vi "send_manipulatorMultiJump-v02.vi"(0 "daq_ao 2":tag="Dev1/ao1", 1 "Duration (s)":dbl, 2 "controls array in":refnum<vi>[](array[refnum]), 3 "Sample Freq (Hz)":dbl min=0.0 max=40000.0, 4 "Delay":dbl, 5 "Position Dwell Time (s)":dbl[](array[numeric]), 6 "daq_ai":tag="Dev1/ai0:1", 8 "Use Current Position for Start Pos?":bool, 9 "Number of Replicates":i16=1 min=1 max=10, 10 "Start Position":T4(ring)=enum."Jumper Position C", 11 "common cluster":T5, 12 "Jump Position Array":T3(array[ring]), 13 "error in":errorcluster) -> (14 "output cluster":T1, 16 "control array out":refnum<vi>[](array[refnum]), 17 "protcol waveform":waveform(dbl)(graph), 18 "error out":errorcluster, 19 "protcol response":waveform(dbl)[](graph) caption="jumptestMonitor")   [LabVIEW 2019]
uses:
  multipatch/controls/multipatch_common_controls_v4.ctl
  machine_vision/controls/transform_cluster_actuator.ctl
  machine_vision/coordinate model vis/transform_properties_actuators.ctl
  pipette cleaning/pressure box/cleaning_soft/controls/actuator_cluster.ctl
  pipette cleaning/pressure box/cleaning_soft/controls/actuator_type.ctl
  pipette cleaning/pressure box/cleaning_soft/controls/pressure_box_control.ctl
  pipette cleaning/pressure box/cleaning_soft/controls/pressure_box_type.ctl
  controls/NH_method.ctl
  <vilib>/measure/NI_MABase.lvlib
panel:
  out "PositionClusterArray":T2(array[cluster])
  in  "Jump Filter Freq (Hz)":dbl=20.0 min=0.0 max=40000.0
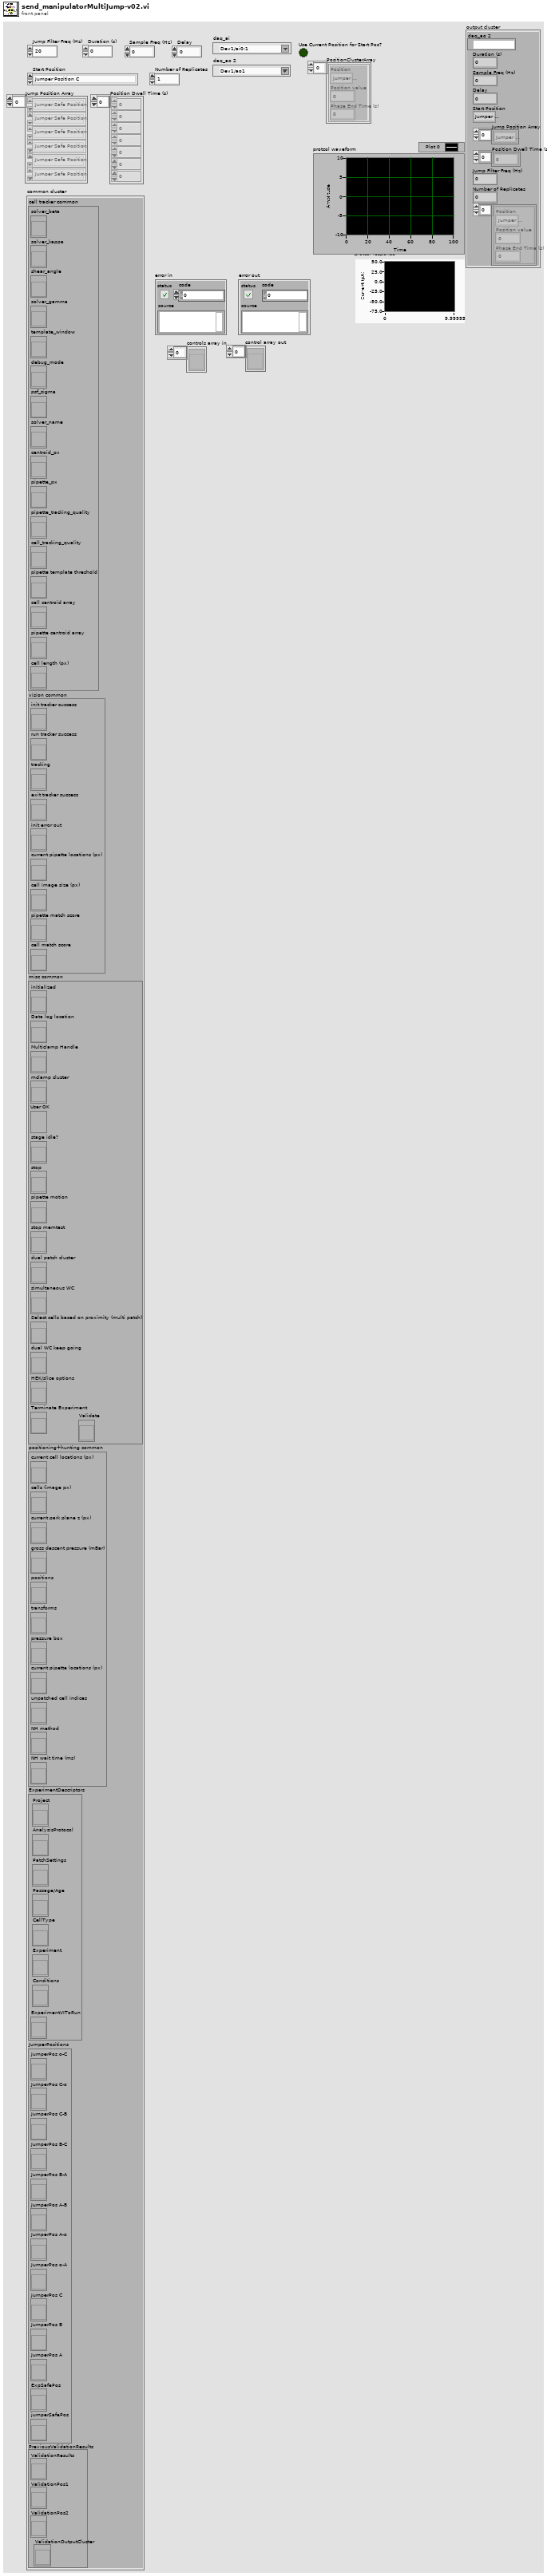
[diagram p1: front panel]
types:
  T1 = cluster{"daq_ao 2":tag, "Duration (s)":dbl, "Sample Freq (Hz)":dbl, "Delay":dbl, "Start Position":enum16{"Jumper Safe Position", "Experiment Safe Position", "Jumper Position A", "Jumper Position B", "Jumper Position C", "Jumper Position o-A", "Jumper Position A-o", "Jumper Position A-B", "Jumper Position B-A", "Jumper Position B-C", "Jumper Position C-B", "Jumper Position C-o", "Jumper Position o-C"}, "Jump Position Array":enum16{"Jumper Safe Position", "Experiment Safe Position", "Jumper Position A", "Jumper Position B", "Jumper Position C", "Jumper Position o-A", "Jumper Position A-o", "Jumper Position A-B", "Jumper Position B-A", "Jumper Position B-C", "Jumper Position C-B", "Jumper Position C-o", "Jumper Position o-C"}[], "Position Dwell Time (s)":dbl[], "Jump Filter Freq (Hz)":dbl, "Number of Replicates":i16, cluster{"Position":enum16{"Jumper Safe Position", "Experiment Safe Position", "Jumper Position A", "Jumper Position B", "Jumper Position C", "Jumper Position o-A", "Jumper Position A-o", "Jumper Position A-B", "Jumper Position B-A", "Jumper Position B-C", "Jumper Position C-B", "Jumper Position C-o", "Jumper Position o-C"}, "Position value":i32, "Phase End Time (s)":dbl}[]}
  T2 = cluster{"Position":enum16{"Jumper Safe Position", "Experiment Safe Position", "Jumper Position A", "Jumper Position B", "Jumper Position C", "Jumper Position o-A", "Jumper Position A-o", "Jumper Position A-B", "Jumper Position B-A", "Jumper Position B-C", "Jumper Position C-B", "Jumper Position C-o", "Jumper Position o-C"}, "Position value":i32, "Phase End Time (s)":dbl}[]
  T3 = enum16{"Jumper Safe Position", "Experiment Safe Position", "Jumper Position A", "Jumper Position B", "Jumper Position C", "Jumper Position o-A", "Jumper Position A-o", "Jumper Position A-B", "Jumper Position B-A", "Jumper Position B-C", "Jumper Position C-B", "Jumper Position C-o", "Jumper Position o-C"}[]
  T4 = enum16{"Jumper Safe Position", "Experiment Safe Position", "Jumper Position A", "Jumper Position B", "Jumper Position C", "Jumper Position o-A", "Jumper Position A-o", "Jumper Position A-B", "Jumper Position B-A", "Jumper Position B-C", "Jumper Position C-B", "Jumper Position C-o", "Jumper Position o-C"}
  T5 = typedef "multipatch_common_controls_v4.ctl" = cluster{"cell tracker common":cluster{"solver_beta":refnum<vi>, "solver_kappa":refnum<vi>, "shear_angle":refnum<vi>, "solver_gamma":refnum<vi>, "template_window":refnum<vi>, "debug_mode":refnum<vi>, "psf_sigma":refnum<vi>, "solver_name":refnum<vi>, "centroid_px":refnum<vi>, "pipette_px":refnum<vi>, "pipette_tracking_quality":refnum<vi>, "cell_tracking_quality":refnum<vi>, "pipette template threshold":refnum<vi>, "cell centroid array":refnum<vi>, "pipette centroid array":refnum<vi>, "cell length (px)":refnum<vi>}, "vision common":cluster{"init tracker success":refnum<vi>, "run tracker success":refnum<vi>, "tracking":refnum<vi>, "exit tracker success":refnum<vi>, "init error out":refnum<vi>, "current pipette locations (px)":refnum<vi>, "cell image size (px)":refnum<vi>, "pipette match score":refnum<vi>, "cell match score":refnum<vi>}, "misc common":cluster{"initialized":refnum<vi>, "Data log location":refnum<vi>, "Multiclamp Handle":refnum<vi>, "mclamp cluster":refnum<vi>, "User OK":refnum<vi>, "stage idle?":refnum<vi>, "stop":refnum<vi>, "pipette motion":refnum<vi>, "stop memtest":refnum<vi>, "dual patch cluster":refnum<vi>, "simultaneous WC":refnum<vi>, "Select cells based on proximity (multi patch)":refnum<vi>, "dual WC keep going":refnum<vi>, "HEK/slice options":refnum<vi>, "Terminate Experiment":refnum<vi>, "Validate":refnum<vi>}, "positioning+hunting common":cluster{"current cell locations (px)":refnum<vi>, "cells (image px)":refnum<vi>, "current park plane z (px)":refnum<vi>, "gross descent pressure (mBar)":refnum<vi>, "positions":refnum<vi>, "transforms":refnum<vi>, "pressure box":refnum<vi>, "current pipette locations (px)":refnum<vi>, "unpatched cell indices":refnum<vi>, "NH method":refnum<vi>, "NH wait time (ms)":refnum<vi>}, "ExperimentDescriptors":cluster{"Project":refnum<vi>, "AnalysisProtocol":refnum<vi>, "PatchSettings":refnum<vi>, "Passage/Age":refnum<vi>, "CellType":refnum<vi>, "Experiment":refnum<vi>, "Conditions":refnum<vi>, "ExperimentVIToRun":refnum<vi>}, "JumperPositions":cluster{"JumperPos o-C":refnum<vi>, "JumperPos C-o":refnum<vi>, "JumperPos C-B":refnum<vi>, "JumperPos B-C":refnum<vi>, "JumperPos B-A":refnum<vi>, "JumperPos A-B":refnum<vi>, "JumperPos A-o":refnum<vi>, "JumperPos o-A":refnum<vi>, "JumperPos C":refnum<vi>, "JumperPos B":refnum<vi>, "JumperPos A":refnum<vi>, "ExpSafePos":refnum<vi>, "jumperSafePos":refnum<vi>}, "PreviousValidationResults":cluster{"ValidationResults":refnum<vi>, "ValidationPos1":refnum<vi>, "ValidationPos2":refnum<vi>, "ValidationOutputCluster":refnum<vi>}}
  T6 = cluster{"Position":enum16{"Jumper Safe Position", "Experiment Safe Position", "Jumper Position A", "Jumper Position B", "Jumper Position C", "Jumper Position o-A", "Jumper Position A-o", "Jumper Position A-B", "Jumper Position B-A", "Jumper Position B-C", "Jumper Position C-B", "Jumper Position C-o", "Jumper Position o-C"}, "Position value":i32, "Phase End Time (s)":dbl}
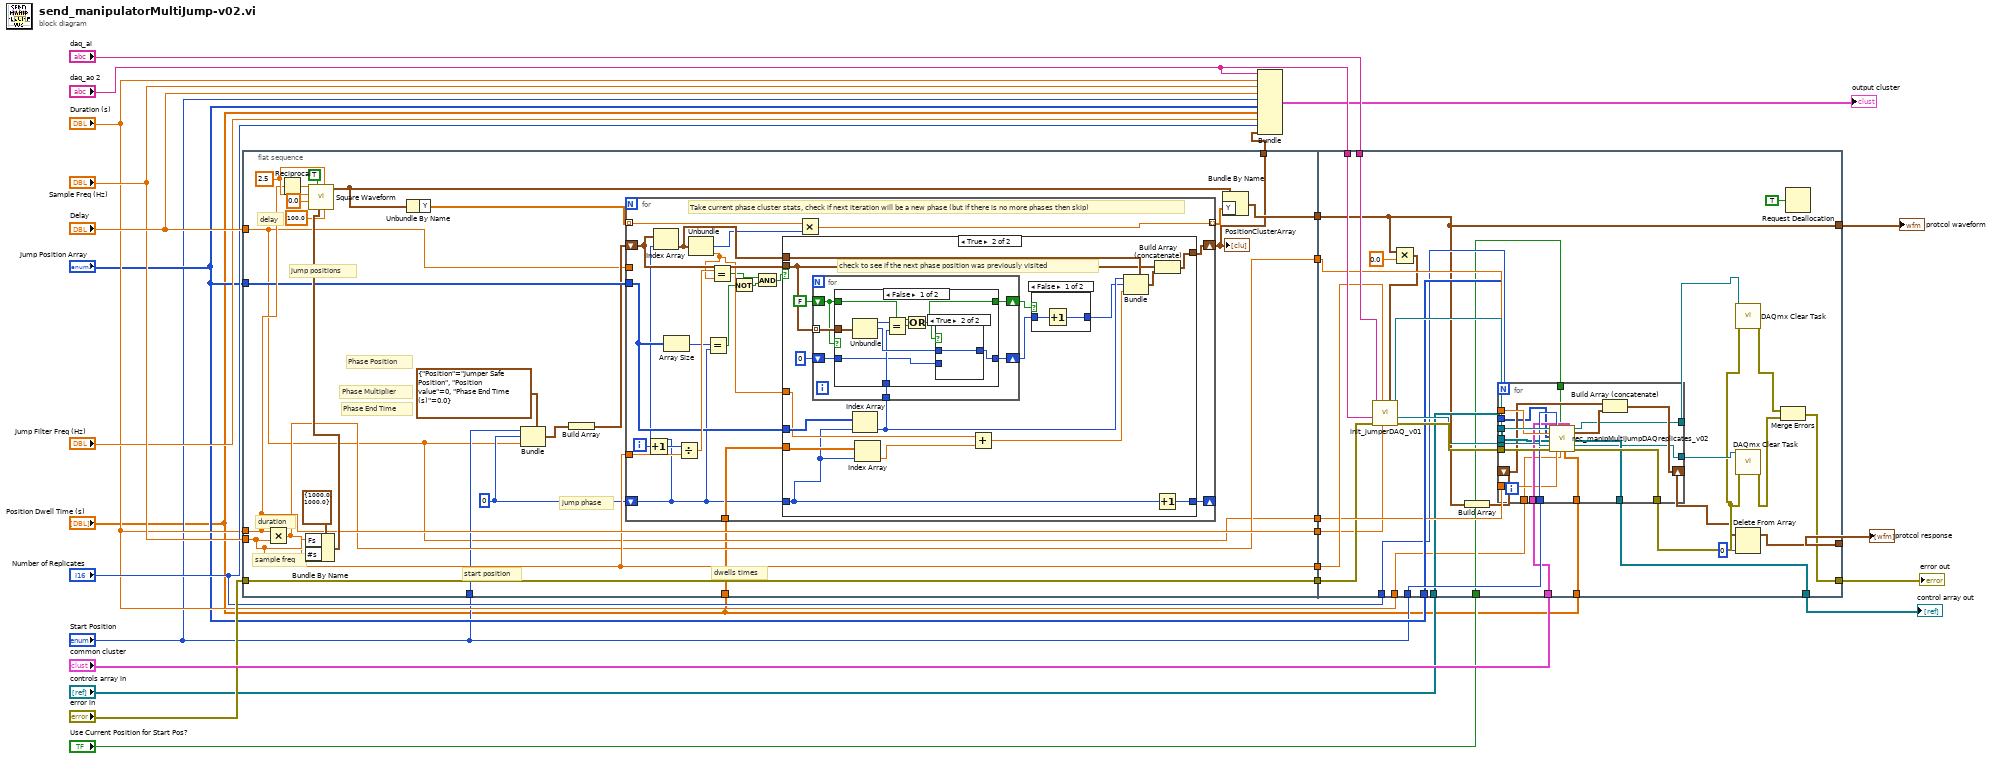
[diagram p0: block diagram]
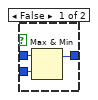
[diagram p4: hidden frame]
diagram:
  n1 = flat-sequence {
    tunnel: "Delay" -> [w30]
    tunnel: "Duration (s)" -> [w44]
    tunnel: "Sample Freq (Hz)" -> [w37]
    tunnel: [w36] -> w20
    tunnel: [w37] -> w18
    tunnel: [w40] -> w19
    tunnel: "error in" -> [w45]
    tunnel: [w45] -> w15
    tunnel: [w44] -> w8
    tunnel: [w30] -> w5
    tunnel: "Jump Position Array" -> [w35]
    tunnel: "Start Position" -> [w34]
    tunnel: "Position Dwell Time (s)" -> [w29]
    tunnel: [w27] -> w1
    tunnel: [w117] -> w25
    tunnel: w20 -> [w140]
    tunnel: w19 -> [w117]
    tunnel: "daq_ai" -> [w143]
    tunnel: "daq_ao 2" -> [w142]
    tunnel: w18 -> [w141]
    tunnel: [w121] -> w22
    tunnel: "Number of Replicates" -> [w131]
    tunnel: "Start Position" -> [w137]
    tunnel: "Jump Position Array" -> [w136]
    tunnel: "common cluster" -> [w135]
    tunnel: [w125] -> w14
    tunnel: w15 -> [w130]
    tunnel: "controls array in" -> [w133]
    tunnel: [w132] -> w12
    tunnel: w8 -> [w119]
    tunnel: "Use Current Position for Start Pos?" -> [w118]
    tunnel: "Duration (s)" -> [w116]
    tunnel: "Position Dwell Time (s)" -> [w115]
    tunnel: w5 -> [w134]
    frame #0 {
      w33 = 0
      w50 = 2.5 ("Amplitude")
      # "dwells times"
      # "start position"
      # "duration"
      # "sample freq"
      # "jump positions"
      # "delay"
      # "Phase End Time"
      # "Phase Multiplier"
      # "Phase Position"
      # "jump phase"
      n2 = Multiply(x=w44, y=w37) -> (x*y=w36:dbl)
      n3 = Reciprocal(x=w44) -> (1/x=w46:dbl)
      n4 = Bundle By Name(cluster=cluster{"Fs":dbl, "#s":dbl} {"Fs"=1000.0, "#s"=1000.0} ("sampling info"), "Fs"=w37, "#s"=w36) -> (w47:cluster{"Fs":dbl, "#s":dbl})
      n5 = call <vilib>:"Square Waveform.vi"("duty cycle (%)"=100.0, "offset"=w50, "sampling info"=w47, "reset signal"=TRUE, "phase"=0.0, "amplitude"=w50, "frequency"=w46) -> ("signal out"=w41:waveform(dbl))  [unwired: 3 in, 1 out]
      n6 = Unbundle By Name(w41) -> ("Y"=w39:dbl[])
      n7 = Bundle(cluster=T6 {"Position"=enum."Jumper Safe Position", "Position value"=0, "Phase End Time (s)"=0.0} ("PositionsPhaseCluster"), "Position"=w34, "Position value"=w33, "Phase End Time (s)"=w30) -> (w32:T6)
      n8 = Build Array(w32) -> (w31:T2)
      n9 = for {
        tunnel: w39 -> [w70] mode=indexing
        tunnel: [w67] -> w38 mode=indexing
        tunnel: w37 -> [w68]
        tunnel: w30 -> [_]
        tunnel: w35 -> [w57]
        shift-right: [w66] -> _
        shift-left: w33 -> [w55]
        shift-right: [w62] -> w27
        shift-left: w31 -> [w63]
        tunnel: w29 -> [w58]
        i -> [w69]
        # "Take current phase cluster stats, check if next iteration will be a new phase (but if there is no more phases then skip)"
        n10 = Increment(x=w69) -> (x+1=w65:i32)
        n11 = Index Array(array=w63, index=w55) -> (element=w61:T6)
        n12 = Array Size(array=w57) -> (size(s)=w56:i32)
        n13 = Divide(x=w65, y=w68) -> (x/y=w64:dbl)
        n14 = Unbundle(w61) -> ("Position value"=w59:i32, "Phase End Time (s)"=w60:dbl)  [unwired: 1 out]
        n15 = Equal?(x=w56, y=w55) -> (x = y?=w52:bool)
        n16 = Equal?(x=w64, y=w60) -> (x = y?=w53:bool)
        n17 = Not(x=w52) -> (.not. x?=w51:bool)
        n18 = And(x=w53, y=w51) -> (x .and. y?=w54:bool)
        n19 = case shown="True" w54 {
          tunnel: w55 -> [w72 w73]
          tunnel: [w72 w89] -> w66
          tunnel: w63 -> [w71 w80]
          tunnel: [w71 w88] -> w62
          tunnel: w61 -> [_ w87]
          tunnel: w60 -> [_ w83]
          tunnel: w57 -> [_ w85]
          tunnel: w58 -> [_ w84]
          frame False {
          }
          frame True {
            # "check to see if the next phase position was previously visited"
            n20 = Index Array(array=w85, index=w73) -> (element=w79:T4)
            n21 = for {
              tunnel: w80 -> [w98] mode=indexing
              tunnel: w79 -> [w96]
              shift-right: [w97] -> w75
              shift-left: 0 -> [w95]
              shift-right: [w94] -> w77
              shift-left: FALSE ("x = y?") -> [w93]
              n22 = case shown="False" w93 {
                tunnel: w98 -> [w107 _]
                tunnel: [w105 w112] -> w97
                tunnel: w96 -> [w103 _]
                tunnel: w95 -> [w102 w112]
                tunnel: w93 -> [w100 w113]
                tunnel: [w99 w113] -> w94
                frame False {
                  n23 = Unbundle(w107) -> ("Position"=w104:T4, "Position value"=w106:i32)  [unwired: 1 out]
                  n24 = Equal?(x=w104, y=w103) -> (x = y?=w101:bool)
                  n25 = Or(x=w100, y=w101) -> (x .or. y?=w99:bool)
                  n26 = case shown="True" w99 {
                    tunnel: w106 -> [w109 w111]
                    tunnel: [w108 w111] -> w105
                    tunnel: w102 -> [w110 _]
                    frame False {
                      n27 = Max & Min(x=w109, y=w110) -> (max(x,y)=w108:i32)  [unwired: 1 out]
                    }
                    frame True {
                    }
                  }
                }
                frame True {
                }
              }
            }
            n28 = Index Array(array=w84, index=w73) -> (element=w81:dbl)
            n29 = Add(x=w83, y=w81) -> (x+y=w82:dbl)
            n30 = case shown="False" w77 {
              tunnel: w75 -> [w91 w92]
              tunnel: [w90 w92] -> w76
              frame False {
                n31 = Increment(x=w91) -> (x+1=w90:i32)
              }
              frame True {
              }
            }
            n32 = Bundle(cluster=w87, "Position"=w79, "Position value"=w76, "Phase End Time (s)"=w82) -> (w86:T6)
            n33 = Build Array (concatenate)(w80, w86) -> (w88:T2)
            n34 = Increment(x=w73) -> (x+1=w89:i32)
          }
        }
        n35 = Multiply(x=w70, y=w59) -> (x*y=w67:dbl)
      }
      "PositionClusterArray" <- w27
      n36 = Bundle By Name(cluster=w41, "Y"=w38) -> (w40:waveform(dbl))
    }
    frame #1 {
      n37 = Multiply(x=w117, y=0.0) -> (x*y=w138:waveform(dbl))
      n38 = call "init_jumperDAQ_v01.vi"("protocol waveform"=w138, "Duration (s)"=w119, "Sample Freq (Hz)"=w141, "AO error in"=w130, "AO physical channels"=w142, "AI Physical Channel"=w143) -> ("AO error out"=w146:errorcluster, "AO task out"=w145:refnum<k21>, "AI task out"=w144:refnum<k21>)  [unwired: 1 in, 2 out]
      n39 = Build Array(w117) -> (w123:waveform(dbl)[])
      n40 = for {
        N: w131 -> [_]
        tunnel: w146 -> [w165]
        tunnel: w145 -> [w164]
        tunnel: w144 -> [w163]
        tunnel: w140 -> [w161]
        tunnel: w137 -> [w160]
        tunnel: w136 -> [w148]
        tunnel: w135 -> [w159]
        tunnel: w134 -> [w158]
        tunnel: w133 -> [w157]
        tunnel: [w156] -> w132
        shift-right: [w155] -> w122
        shift-left: w123 -> [w153]
        tunnel: [w162] -> w127
        tunnel: [w152] -> w129
        tunnel: [w151] -> w128
        tunnel: w116 -> [w150]
        tunnel: w118 -> [w149]
        tunnel: w115 -> [w147]
        n41 = call "rec_manipMultiJumpDAQreplicates_v02.vi"("AI task in"=w163, "number of samples"=w161, "Jump Position Array"=w148, "controls array in"=w157, "AO task in"=w164, "error in"=w165, "Start Position"=w160, "Delay"=w158, "Use Current Position for Start Pos?"=w149, "Duration (s)"=w150, "Position Dwell Time (s)"=w147, "common cluster"=w159) -> ("AI task out"=w151:refnum<k21>, "data out (pA or mV)"=w154:waveform(dbl), "control array out"=w156:refnum<vi>[], "AO task out"=w152:refnum<k21>, "error out"=w162:errorcluster)  [unwired: 3 in]
        n42 = Build Array (concatenate)(w153, w154) -> (w155:waveform(dbl)[])
      }
      n43 = call <vilib>:"DAQmx Clear Task.vi"("task in"=w128, "error in"=w127) -> ("error out"=w124:errorcluster)  [unwired: 13 in]
      n44 = call <vilib>:"DAQmx Clear Task.vi"("task in"=w129, "error in"=w127) -> ("error out"=w126:errorcluster)  [unwired: 13 in]
      n45 = Delete From Array(array=w122, index=0) -> (array with subset deleted=w121:waveform(dbl)[])  [unwired: 1 in, 1 out]
      n46 = Merge Errors(w124, w126) -> (w125:errorcluster)
      n47 = Request Deallocation(TRUE ("flag")) -> ()
    }
  }
  n48 = Bundle("daq_ao 2"="daq_ao 2", "Duration (s)"="Duration (s)", "Sample Freq (Hz)"="Sample Freq (Hz)", "Delay"="Delay", "Start Position"="Start Position", "Jump Position Array"="Jump Position Array", "Position Dwell Time (s)"="Position Dwell Time (s)", "Jump Filter Freq (Hz)"="Jump Filter Freq (Hz)", "Number of Replicates"="Number of Replicates", w1) -> (→"output cluster":T1)  [unwired: 1 in]
  "protcol response" <- w22
  "protcol waveform" <- w25
  "error out" <- w14
  "control array out" <- w12
